vi "set_settings_value.vi"(8 "error in (no error)":errorcluster, 9 "value":u16, 10 "SETTINGS_Cmd":T1, 11 "TCP Network Connection in":refnum<k5>) -> (0 "error out":errorcluster, 2 "success?":bool, 3 "TCP Network Connection out":refnum<k5>)   [LabVIEW 2021]
uses:
  typedefs/SETTINGS_Cmd.ctl
  typedefs/w5500_cmd.ctl
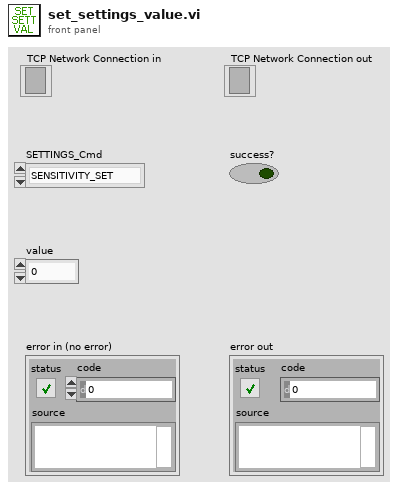
[diagram p1: front panel]
types:
  T1 = typedef "SETTINGS_Cmd.ctl" = enum8{"SENSITIVITY_SET", "SENSITIVITY_VAL", "RECORD_TIME_SET", "RECORD_TIME_VAL", "DISC_FREQ_SET", "DISC_FREQ_VAL", "STATE_SET", "STATE_VAL"}
  T2 = typedef "w5500_cmd.ctl" = enum32{"LAN_TRANS_START", "LAN_DATA_SZ", "LAN_CHUNK_SEND", "LAN_CHUNK_ACK", "LAN_DEVS_INFO", "LAN_DEVS_NUM", "LAN_DEVS_EXS", "LAN_DEVS_ACK", "LAN_CMD_ACK", "LAN_CMD_FIN", "LAN_SND_STAT", "LAN_REQ_STAT", "LAN_ANS_STAT", "LAN_ERR_STAT", "LAN_SETT_SET", "LAN_SETT_GET", "LAN_SETT_ACK", "LAN_SETT_ERR"}
  T3 = typedef "SETTINGS_Pck.ctl" = cluster{"SETTINGS_Cmd":T1, "_pad":u8, "val_sett":u16}
  T4 = typedef "w5500_pck.ctl" = cluster{"cmd_type":T2, "pck_num":u32, "dev_id":u32, "data":u8[]}
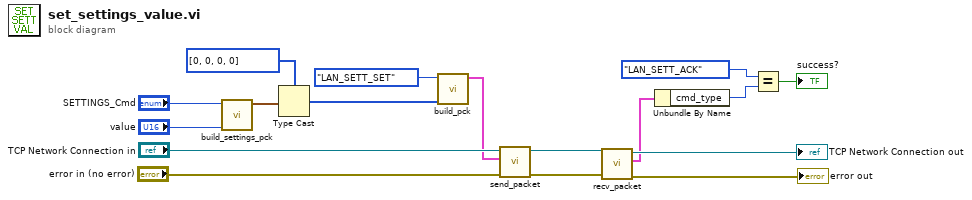
[diagram p0: block diagram]
diagram:
  n1 = call "build_settings_pck.vi"("value"="value", "SETTINGS_Cmd"="SETTINGS_Cmd") -> ("SETTINGS_Pck"=w4:T3)  [unwired: 9 in]
  n2 = Type Cast(type=u8[] [0, 0, 0, 0] ("data in"), x=w4) -> (*(type *) &x=w6:u8[])
  n3 = call "build_pck.vi"("data in"=w6, "cmd_type"=w5500_cmd."LAN_SETT_SET") -> ("w5500_pck"=w7:T4)  [unwired: 9 in]
  n4 = call "send_packet.vi"("error in (no error)"="error in (no error)", "w5500_pck in"=w7, "TCP Network Connection in"="TCP Network Connection in") -> ("error out"=w11:errorcluster, "TCP Network Connection out"=w10:refnum<k5>)  [unwired: 7 in]
  n5 = call "recv_packet.vi"("error in (no error)"=w11, "TCP Network Connection in"=w10) -> ("error out"=→"error out":errorcluster, "w5500_pck"=w12:T4, "TCP Network Connection out"=→"TCP Network Connection out":refnum<k5>)  [unwired: 7 in]
  n6 = Unbundle By Name(w12) -> ("cmd_type"=w13:T2)
  n7 = Equal?(x=w5500_cmd."LAN_SETT_ACK" ("cmd_type"), y=w13) -> (x = y?=→"success?":bool)
